vi "加减计数器.vi"(6 "reset":bool, 7 "load":bool, 8 "error in":errorcluster, 9 "preset value":u32=10, 10 "count down":bool, 11 "count up":bool) -> (0 "error out":errorcluster, 1 "counter value":u32, 2 "count down done":bool, 3 "count up done":bool)   [LabVIEW 2013]
uses:
  <vilib>/ptbypt/NI_PtbyPt.lvlib
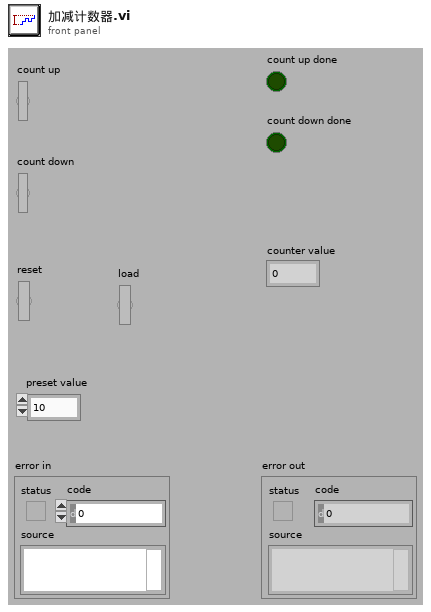
[diagram p1: front panel]
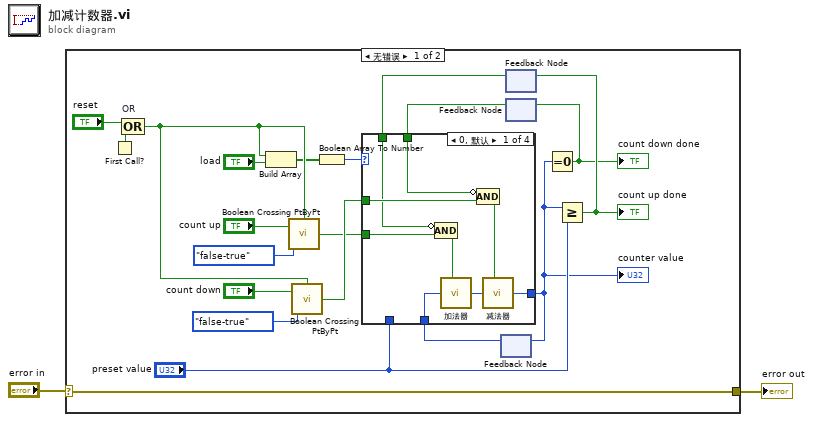
[diagram p0: block diagram]
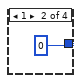
[diagram p2: hidden frame]
diagram:
  n1 = case shown="无错误" "error in" {
    selector: "error in" -> [w22 w35]
    tunnel: [w22 w35] -> w1
    frame No Error {
      n2 = First Call?() -> (First Call?: T/F=w20:bool)
      n3 = Compound Arithmetic op=OR "OR"("reset", w20) -> (w6:bool)
      n4 = Build Array(w6, "load") -> (w4:bool[])
      n5 = call <vilib>:"Boolean Crossing PtByPt.vi"("initialize"=w6, "direction"=enum16{"either", "false-true", "true-false"}."false-true", "input"="count up") -> ("crossing"=w11:bool)
      n6 = call <vilib>:"Boolean Crossing PtByPt.vi"("initialize"=w6, "direction"=enum16{"either", "false-true", "true-false"}."false-true", "input"="count down") -> ("crossing"=w13:bool)
      n7 = Boolean Array To Number(Boolean array=w4) -> (number=w3:u32)
      n8 = feedback #1() -> (w15:u32)  [unwired: 1 in]
      n9 = feedback #2() -> (w12:bool)  [unwired: 1 in]
      n10 = feedback #3() -> (w14:bool)  [unwired: 1 in]
      n11 = case shown="0, 默认" w3 {
        tunnel: [w25 u32 0 w33 w34] -> w7
        tunnel: w15 -> [w26 _ _ _]
        tunnel: w11 -> [w28 _ _ _]
        tunnel: w13 -> [w27 _ _ _]
        tunnel: w14 -> [w23 _ _ _]
        tunnel: w12 -> [w24 _ _ _]
        tunnel: "preset value" -> [_ _ w33 w34]
        frame 0, Default {
          n12 = Compound Arithmetic op=AND ("AND")(invert w24, w28) -> (w31:bool)
          n13 = call-poly "加法器.vi"("Enable(T)"=w31, "In"=w26) -> ("Out"=w30:u32)  [unwired: 5 in]
          n14 = Compound Arithmetic op=AND ("AND")(invert w23, w27) -> (w29:bool)
          n15 = call-poly "减法器.vi"("Enable(T)"=w29, "In"=w30) -> ("Out"=w25:u32)  [unwired: 5 in]
        }
        frame 1 {
        }
        frame 2 {
        }
        frame 3 {
        }
      }
      "counter value" <- w7
      n16 = feedback-in #1(w7) -> ()
      n17 = Equal To 0?(x=w7) -> (x = 0?=w8:bool)
      "count down done" <- w8
      n18 = feedback-in #3(w8) -> ()
      n19 = Greater Or Equal?(x=w7, y="preset value") -> (x >= y?=w9:bool)
      "count up done" <- w9
      n20 = feedback-in #2(w9) -> ()
    }
    frame Error {
    }
  }
  "error out" <- w1
